vi "DCp0_2024.vi"(8 "CO2 content (ppm)":dbl=542.0, 9 "molar fraction of water vapor":dbl=0.013091059810824573 format="%.6f", 10 "Temperature / K":dbl=293.4405 format="%.4g", 11 "Type of air":i32(listbox)=4) -> (1 "rel. unc. Cp0 humid air":dbl=0.0002346561264646301 format="%.2e", 2 "rel. unc. Cp0/R water":dbl=0.001 format="%.2e", 3 "rel. unc. Cp0 dry air":dbl=0.0002375951225780895 format="%.2e")   [LabVIEW 2016]
panel:
  out "rel. unc. Cp0 humid air (ppm)":dbl=234.65612646463012 format="%.1f"
  out "rel. unc Cp0/R CO2":dbl=0.001 format="%.2e"
  out "rel. unc. Cp0/R CH4":dbl=0.001 format="%.2e"
  out "relative unc.  monatomic gases":dbl format="%.2e"
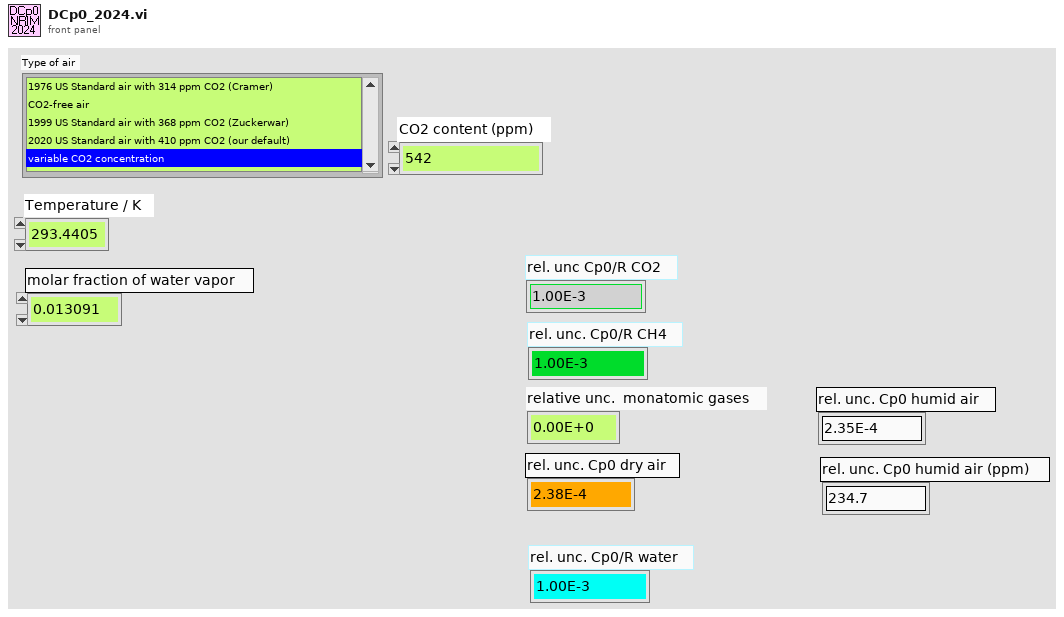
[diagram p1: front panel]
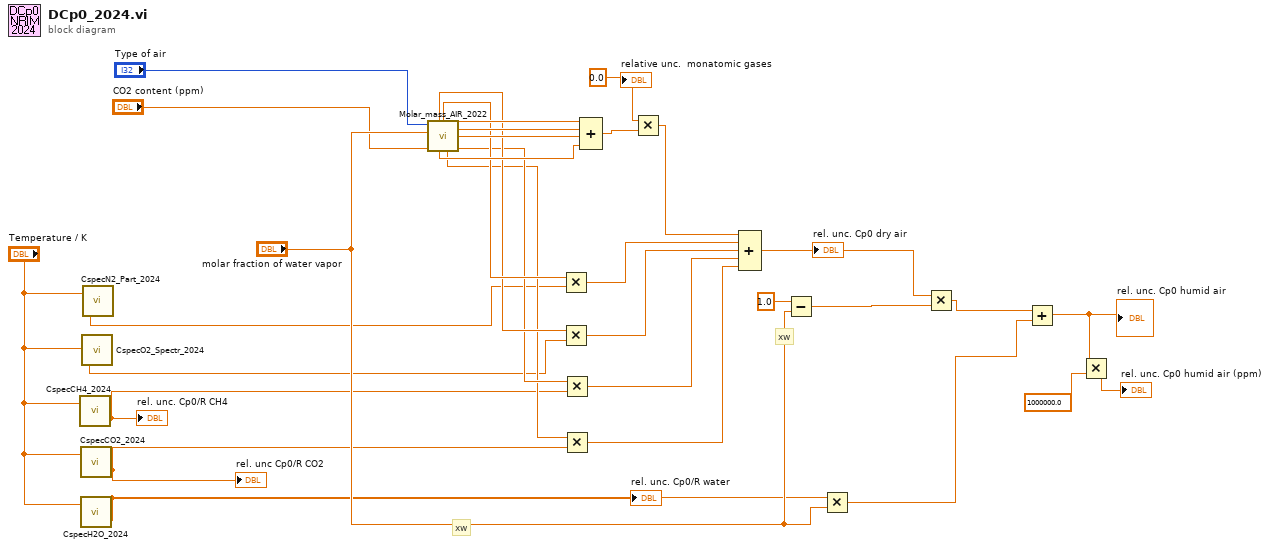
[diagram p0: block diagram]
diagram:
  w1 = 0.0
  # "xw"
  # "xw"
  n1 = call "CspecCH4_2024.vi"("Temperature [K]"="Temperature / K") -> ("rel. unc. Cp0/R CH"=w4:dbl)  [unwired: 4 out]
  "rel. unc. Cp0/R CH4" <- w4
  n2 = call "CspecCO2_2024.vi"("Temperature [K]"="Temperature / K") -> ("rel. unc Cp0/R CO2"=w3:dbl)  [unwired: 4 out]
  "rel. unc Cp0/R CO2" <- w3
  n3 = call "CspecH2O_2024.vi"("Temperature [K]"="Temperature / K") -> ("rel. unc. Cp0/R water"=w5:dbl)  [unwired: 4 out]
  "rel. unc. Cp0/R water" <- w5
  n4 = call "CspecO2_Spectr_2024.vi"("Temperature [K]"="Temperature / K") -> ("rel unc Cp0 O2"=w6:dbl)  [unwired: 4 out]
  n5 = call "CspecN2_Part_2024.vi"("Temperature [K]"="Temperature / K") -> ("rel unc Cp0 N2"=w7:dbl)  [unwired: 4 out]
  n6 = call "Molar_mass_AIR_2022.vi"("CO2 content (ppm)"="CO2 content (ppm)", "xw molar fraction of water vapor"="molar fraction of water vapor", "Type of air"="Type of air") -> ("xCH4"=w26:dbl, "xKr"=w30:dbl, "xHe"=w31:dbl, "xNe"=w32:dbl, "xCO2"=w11:dbl, "xN2"=w28:dbl, "xAr"=w29:dbl, "xO2"=w27:dbl)  [unwired: 1 out]
  n7 = Multiply(x=w28, y=w7) -> (x*y=w23:dbl)
  n8 = Multiply(x=w27, y=w6) -> (x*y=w22:dbl)
  n9 = Multiply(x=w26, y=w4) -> (x*y=w21:dbl)
  n10 = Multiply(x=w11, y=w3) -> (x*y=w20:dbl)
  n11 = Compound Arithmetic op=ADD(w32, w31, w30, w29) -> (w25:dbl)
  n12 = Multiply(x=w1, y=w25) -> (x*y=w24:dbl)
  n13 = Compound Arithmetic op=ADD(w24, w23, w22, w21, w20) -> (w14:dbl)
  "rel. unc. Cp0 dry air" <- w14
  n14 = Subtract(x=1.0, y="molar fraction of water vapor") -> (x-y=w17:dbl)
  n15 = Multiply(x=w5, y="molar fraction of water vapor") -> (x*y=w18:dbl)
  n16 = Multiply(x=w14, y=w17) -> (x*y=w19:dbl)
  n17 = Add(x=w19, y=w18) -> (x+y=w10:dbl)
  "rel. unc. Cp0 humid air" <- w10
  n18 = Multiply(x=w10, y=1000000.0) -> (x*y=→"rel. unc. Cp0 humid air (ppm)":dbl)
  "relative unc.  monatomic gases" <- w1
